vi "Read Lock-In Stream.vi"(7 "instance":i32, 8 "error in":errorcluster, 11 "lia rt in":refnum<class "Lock-In Amplifier Example RT.lvclass">) -> (0 "error out":errorcluster, 3 "lia rt out":refnum<class "Lock-In Amplifier Example RT.lvclass">)   [LabVIEW 2017, in "Lock-In Amplifier Example RT.lvclass"]
uses:
  Lock-In Amplifier Example RT.lvclass
  shared/Public/message.ctl
  Properties/FpgaSession_GET.vi
  interface/Interface FPGA/LIA Host Interface FPGA.lvclass
  shared/Lock-In Amplifier Example Shared.lvlib
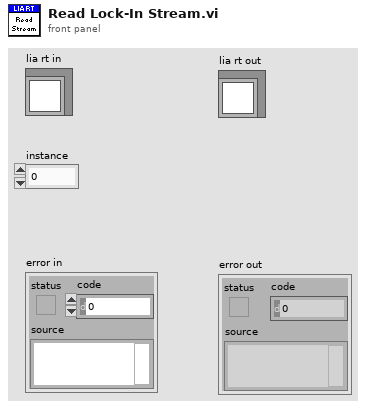
[diagram p1: front panel]
types:
  T1 = typedef "Lock-In Amplifier Example Shared.lvlib/message.ctl" = cluster{"command":u32, "payload":string}
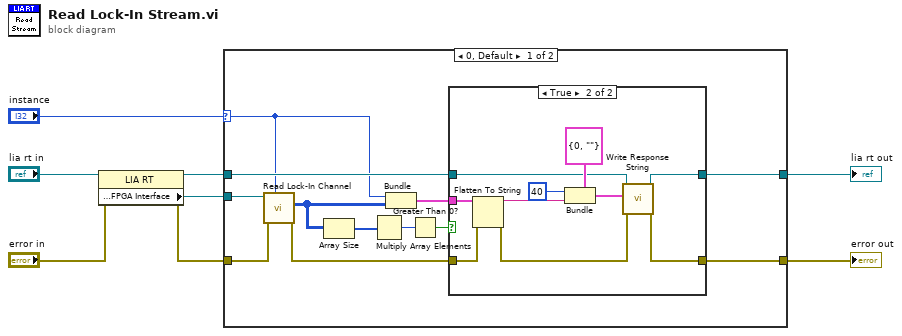
[diagram p0: block diagram]
diagram:
  n1 = property class="LIA RT"(reference="lia rt in", error in="error in") -> (reference out=w3:refnum<class "Lock-In Amplifier Example RT.lvclass">, error out=w5:errorcluster, "Properties:FPGA Interface"=w4:refnum<class "LIA Host Interface FPGA.lvclass">)
  n2 = case shown="0, Default" "instance" {
    selector: "instance" -> [w13 _]
    tunnel: w4 -> [w17 _]
    tunnel: w5 -> [w16 w34]
    tunnel: w3 -> [w15 w33]
    tunnel: [w20 w33] -> w2
    tunnel: [w19 w34] -> w1
    frame 0, Default {
      n3 = call-dynamic "Read Lock-In Channel.vi"("index"=w13, "error in"=w16, "host in"=w17) -> ("error out"=w14:errorcluster, "unscaled data"=w12:i64[][])  [unwired: 6 in, 1 out]
      n4 = Array Size(array=w12) -> (size(s)=w11:i32[])
      n5 = Multiply Array Elements(1:w11) -> (0:w10:i32)
      n6 = Bundle("instance"=w13, "unscaled data"=w12) -> (w18:cluster{"instance":i32, "unscaled data":i64[][]})  [unwired: 1 in]
      n7 = Greater Than 0?(x=w10) -> (x > 0?=w9:bool)
      n8 = case shown="True" w9 {
        tunnel: w18 -> [_ w32]
        tunnel: w14 -> [w21 w31]
        tunnel: [w21 w26] -> w19
        tunnel: w15 -> [w22 w25]
        tunnel: [w22 w24] -> w20
        frame False {
        }
        frame True {
          n9 = Flatten To String(anything=w32, error in (no error)=w31) -> (data string=w23:string, error out=w27:errorcluster)  [unwired: 2 in, 1 out]
          n10 = Bundle(cluster=T1 {"command"=0, "payload"=""} ("message in"), "command"=40, "payload"=w23) -> (w28:T1)
          n11 = call "Write Response String.vi"("error in"=w27, "message in"=w28, "lia rt in"=w25) -> ("error out"=w26:errorcluster, "lia rt out"=w24:refnum<class "Lock-In Amplifier Example RT.lvclass">)  [unwired: 7 in]
        }
      }
    }
    frame 1 {
    }
  }
  "error out" <- w1
  "lia rt out" <- w2
